vi "Camera Get Image.vi"(5 "Xmit":bool, 7 "Network Data":T2, 8 "error in (no error)":errorcluster, 9 "Camera Cluster":cluster{"Session Out":T4, "Camera Number":i32}, 10 "Camera Controls":T5 {"VideoMode" items=["640 x 480 YUY 2 30.00 fps", "640 x 480 YUY 2 20.00 fps", "640 x 480 YUY 2 15.00 fps", "640 x 480 YUY 2 10.00 fps", "640 x 480 YUY 2 7.50 fps", "1280 x 720 YUY 2 10.00 fps", "1280 x 720 YUY 2 7.50 fps", "960 x 544 YUY 2 15.00 fps", "960 x 544 YUY 2 10.00 fps", "960 x 544 YUY 2 7.50 fps", "800 x 448 YUY 2 20.00 fps", "800 x 448 YUY 2 15.00 fps", "800 x 448 YUY 2 10.00 fps", "800 x 448 YUY 2 7.50 fps", "640 x 360 YUY 2 30.00 fps", "640 x 360 YUY 2 20.00 fps", "640 x 360 YUY 2 15.00 fps", "640 x 360 YUY 2 10.00 fps", "640 x 360 YUY 2 7.50 fps", "424 x 240 YUY 2 30.00 fps", "424 x 240 YUY 2 20.00 fps", "424 x 240 YUY 2 15.00 fps", "424 x 240 YUY 2 10.00 fps", "424 x 240 YUY 2 7.50 fps", "352 x 288 YUY 2 30.00 fps", "352 x 288 YUY 2 20.00 fps", "352 x 288 YUY 2 15.00 fps", "352 x 288 YUY 2 10.00 fps", "352 x 288 YUY 2 7.50 fps", "320 x 240 YUY 2 30.00 fps", "320 x 240 YUY 2 20.00 fps", "320 x 240 YUY 2 15.00 fps", "320 x 240 YUY 2 10.00 fps", "320 x 240 YUY 2 7.50 fps", "800 x 600 YUY 2 15.00 fps", "800 x 600 YUY 2 10.00 fps", "800 x 600 YUY 2 7.50 fps", "176 x 144 YUY 2 30.00 fps", "176 x 144 YUY 2 20.00 fps", "176 x 144 YUY 2 15.00 fps", "176 x 144 YUY 2 10.00 fps", "176 x 144 YUY 2 7.50 fps", "160 x 120 YUY 2 30.00 fps", "160 x 120 YUY 2 20.00 fps", "160 x 120 YUY 2 15.00 fps", "160 x 120 YUY 2 10.00 fps", "160 x 120 YUY 2 7.50 fps", "1280 x 800 YUY 2 10.00 fps", "640 x 480 JPEG 30.00 fps", "640 x 480 JPEG 20.00 fps", "640 x 480 JPEG 15.00 fps", "640 x 480 JPEG 10.00 fps", "640 x 480 JPEG 7.50 fps", "1280 x 720 JPEG 30.00 fps", "1280 x 720 JPEG 20.00 fps", "1280 x 720 JPEG 15.00 fps", "1280 x 720 JPEG 10.00 fps", "1280 x 720 JPEG 7.50 fps", "960 x 544 JPEG 30.00 fps", "960 x 544 JPEG 20.00 fps", "960 x 544 JPEG 15.00 fps", "960 x 544 JPEG 10.00 fps", "960 x 544 JPEG 7.50 fps", "800 x 448 JPEG 30.00 fps", "800 x 448 JPEG 20.00 fps", "800 x 448 JPEG 15.00 fps", "800 x 448 JPEG 10.00 fps", "800 x 448 JPEG 7.50 fps", "640 x 360 JPEG 30.00 fps", "640 x 360 JPEG 20.00 fps", "640 x 360 JPEG 15.00 fps", "640 x 360 JPEG 10.00 fps", "640 x 360 JPEG 7.50 fps", "800 x 600 JPEG 30.00 fps", "800 x 600 JPEG 20.00 fps", "800 x 600 JPEG 15.00 fps", "800 x 600 JPEG 10.00 fps", "800 x 600 JPEG 7.50 fps", "416 x 240 JPEG 30.00 fps", "416 x 240 JPEG 20.00 fps", "416 x 240 JPEG 15.00 fps", "416 x 240 JPEG 10.00 fps", "416 x 240 JPEG 7.50 fps", "352 x 288 JPEG 30.00 fps", "352 x 288 JPEG 20.00 fps", "352 x 288 JPEG 15.00 fps", "352 x 288 JPEG 10.00 fps", "352 x 288 JPEG 7.50 fps", "176 x 144 JPEG 30.00 fps", "176 x 144 JPEG 20.00 fps", "176 x 144 JPEG 15.00 fps", "176 x 144 JPEG 10.00 fps", "176 x 144 JPEG 7.50 fps", "320 x 240 JPEG 30.00 fps", "320 x 240 JPEG 20.00 fps", "320 x 240 JPEG 15.00 fps", "320 x 240 JPEG 10.00 fps", "320 x 240 JPEG 7.50 fps", "160 x 120 JPEG 30.00 fps", "160 x 120 JPEG 20.00 fps", "160 x 120 JPEG 15.00 fps", "160 x 120 JPEG 10.00 fps", "160 x 120 JPEG 7.50 fps"]}, 11 "Refnum in":T1) -> (3 "Refnum out":T1(plugin-control))   [LabVIEW 2016]
uses:
  Camera Settings.ctl
  38 Video Mode.ctl
  <vilib>/userdefined/High Color/IMAQdx.ctl
  TCP Port Control.ctl
  <vilib>/vision/Image Controls.llb/IMAQ Image.ctl
  <vilib>/vision/driver/IMAQdx.llb/IMAQdx Buffer Number Mode.ctl
  <vilib>/vision/driver/NI_Vision_Acquisition_Software.lvlib
  <resource>/objmgr/imaqdx.rc
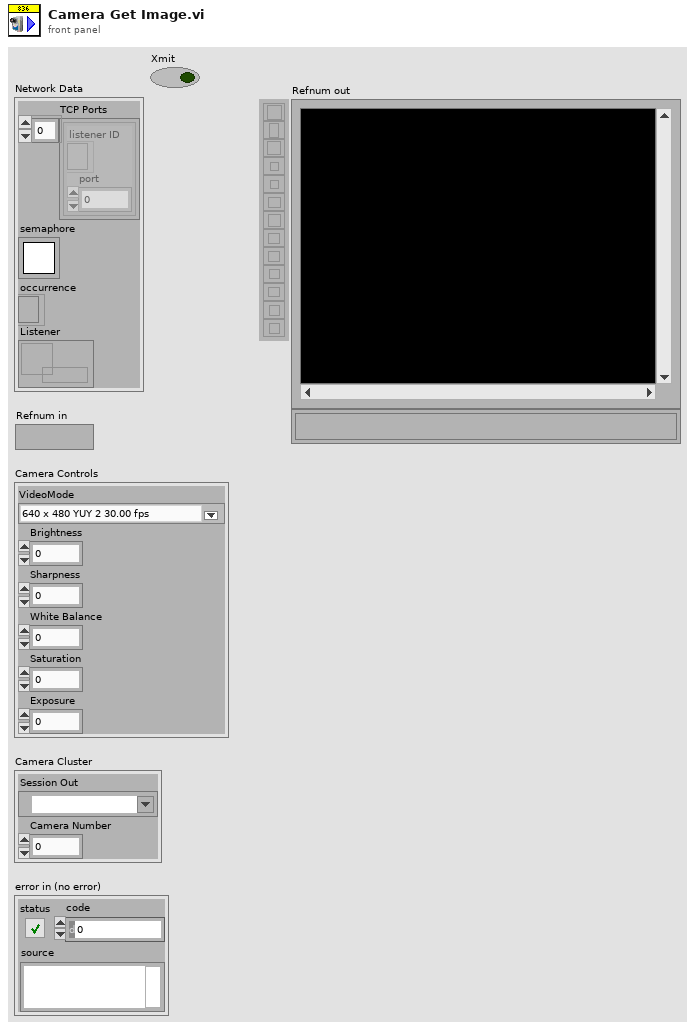
[diagram p1: front panel]
types:
  T1 = typedef "IMAQ Image.ctl" = refnum<image>
  T2 = typedef "TCP Port Control.ctl" = cluster{"TCP Ports":cluster{"listener ID":refnum<k5>, "port":u16}[], "semaphore":T3, "occurrence":refnum<k4>, "Listener":refnum<data-value>}
  T3 = typedef "Semaphore RefNum" = refnum<k1>
  T4 = typedef "IMAQdx.ctl" = refnum<k21>
  T5 = typedef "Camera Settings.ctl" = cluster{"VideoMode":T6, "Brightness":i64, "Sharpness":i64, "White Balance":i64, "Saturation":i64, "Exposure":i64}
  T6 = typedef "38 Video Mode.ctl" = u32
  T7 = typedef "NI_Vision_Acquisition_Software.lvlib/IMAQdx Buffer Number Mode.ctl" = enum32{"Next", "Last", "Buffer Number", "Every", "Last New"}
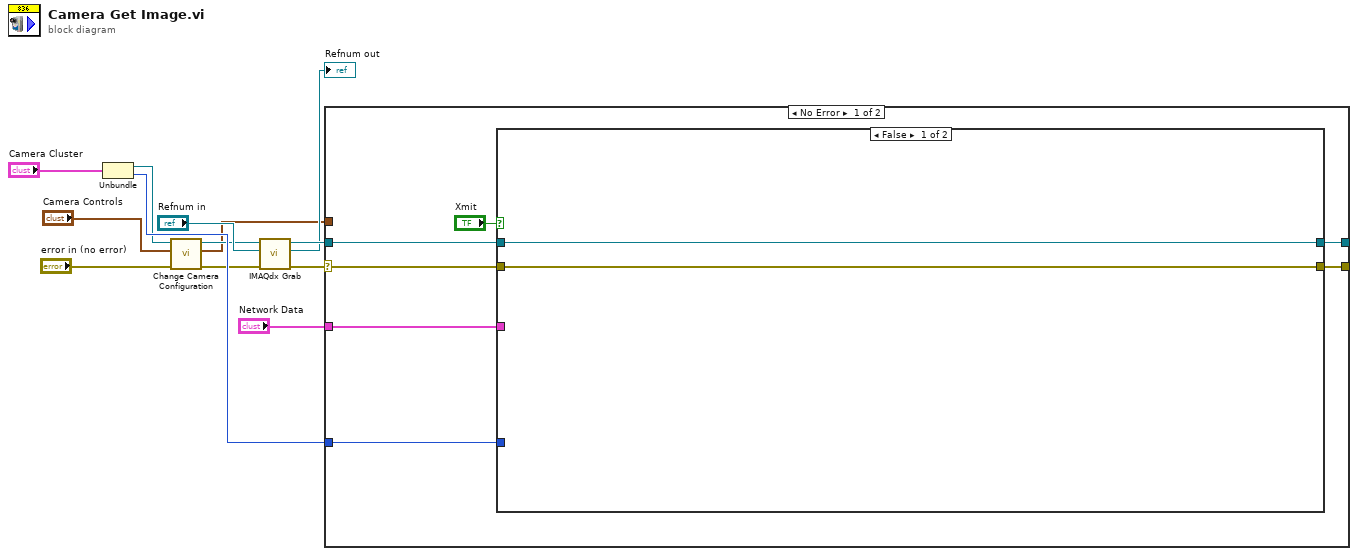
[diagram p0: block diagram]
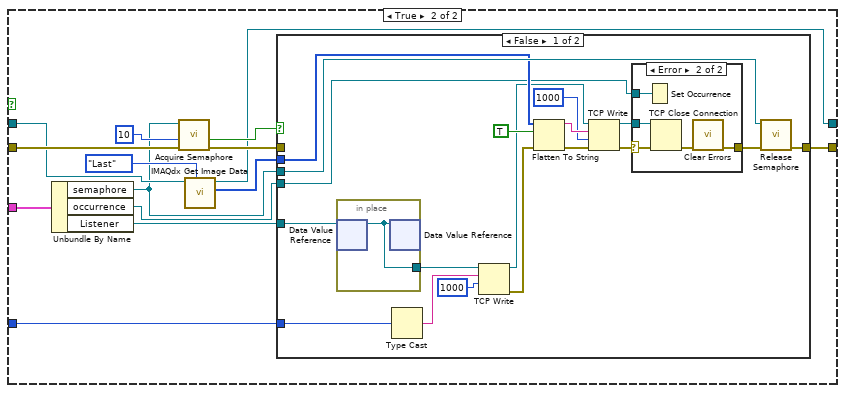
[diagram p2: hidden frame]
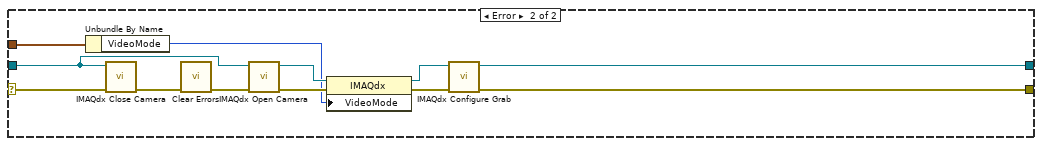
[diagram p5: hidden frame]
diagram:
  n1 = Unbundle("Camera Cluster") -> ("Session Out"=w10:T4, "Camera Number"=w11:i32)
  n2 = call "Change Camera Configuration.vi"("error in (no error)"="error in (no error)", "Camera Controls"="Camera Controls", "Camera Session"=w10) -> ("error out"=w5:errorcluster, "Camera Controls Out"=w1:T5, "Session out"=w2:T4)  [unwired: 6 in]
  n3 = call <vilib>:"IMAQdx Grab.vi"("error in"=w5, "Image In"="Refnum in", "Session In"=w2) -> ("error out"=w6:errorcluster, "Image Out"=→"Refnum out":T1, "Session Out"=w7:T4)  [unwired: 5 in, 1 out]
  n4 = case shown="No Error" w6 {
    selector: w6 -> [w19 w69]
    tunnel: w11 -> [w20 _]
    tunnel: w7 -> [w17 w68]
    tunnel: [w18 w67] -> _
    tunnel: [w16 w66] -> _
    tunnel: w1 -> [_ w63]
    tunnel: "Network Data" -> [w15 _]
    frame No Error {
      n5 = case shown="False" "Xmit" {
        tunnel: w20 -> [_ w34]
        tunnel: w19 -> [w21 w33]
        tunnel: [w21 w32] -> w18
        tunnel: w17 -> [w22 w30]
        tunnel: [w22 w29] -> w16
        tunnel: w15 -> [_ w23]
        frame False {
        }
        frame True {
          n6 = Unbundle By Name(w23) -> ("semaphore"=w24:T3, "occurrence"=w26:refnum<k4>, "Listener"=w25:refnum<data-value>)
          n7 = call <vilib>:"Acquire Semaphore.vi"("error in (no error)"=w33, "ms timeout (-1)"=10, "semaphore"=w24) -> ("error out"=w31:errorcluster, "timed out"=w36:bool)  [unwired: 2 in, 1 out]
          n8 = call <vilib>:"IMAQdx Get Image Data.vi"("Buffer Number Mode (Next)"=IMAQdx_Buffer_Number_Mode."Last", "Session In"=w30) -> ("Image Data Array"=w28:u8[], "Session Out"=w29:T4)  [unwired: 6 in, 2 out]
          n9 = case shown="False" w36 {
            tunnel: w24 -> [w50 _]
            tunnel: w25 -> [w49 _]
            tunnel: w28 -> [w47 _]
            tunnel: w34 -> [w46 _]
            tunnel: w26 -> [w41 _]
            tunnel: [w39 _] -> w32
            tunnel: w31 -> [_ _]
            frame False {
              n10 = in-place {
                in-place-border: [w61] -> w48
                n11 = in-place-dvr #1(w49) -> (w61:refnum<k5>)  [unwired: 1 out]
                n12 = in-place-dvr #1(w61) -> ()  [unwired: 2 out]
              }
              n13 = Type Cast(x=w46) -> (*(type *) &x=w45:string)  [unwired: 1 in]
              n14 = TCP Write(connection ID=w48, data in=w45, 9:1000 ("timeout ms (25000)")) -> (connection ID out=w38:refnum<k5>, error out=w51:errorcluster)  [unwired: 1 in, 1 out]
              n15 = Flatten To String(anything=w47, prepend array or string size? (T)=TRUE, error in (no error)=w51) -> (data string=w53:string, error out=w54:errorcluster)  [unwired: 1 in, 1 out]
              n16 = TCP Write(connection ID=w38, data in=w53, error in (no error)=w54, 9:1000 ("timeout ms (25000)")) -> (connection ID out=w37:refnum<k5>, error out=w42:errorcluster)  [unwired: 1 out]
              n17 = case shown="Error" w42 {
                selector: w42 -> [w55 w58]
                tunnel: w41 -> [_ w60]
                tunnel: [w55 w56] -> w40
                tunnel: w37 -> [_ w59]
                frame No Error {
                }
                frame Error {
                  n18 = Set Occurrence(w60) -> ()
                  n19 = TCP Close Connection(connection ID=w59, error in (no error)=w58) -> (error out=w57:errorcluster)  [unwired: 1 in, 1 out]
                  n20 = call <vilib>:"Clear Errors.vi"("error in (no error)"=w57) -> ("error out"=w56:errorcluster)  [unwired: 5 in, 1 out]
                }
              }
              n21 = call <vilib>:"Release Semaphore.vi"("error in (no error)"=w40, "semaphore"=w50) -> ("error out"=w39:errorcluster)  [unwired: 4 in, 1 out]
            }
            frame True {
            }
          }
        }
      }
    }
    frame Error {
      n22 = Unbundle By Name(w63) -> ("VideoMode"=w62:T6)
      n23 = call <vilib>:"IMAQdx Close Camera.vi"("error in"=w69, "Session In"=w68) -> ("error out"=w73:errorcluster)  [unwired: 9 in]
      n24 = call <vilib>:"Clear Errors.vi"("error in (no error)"=w73) -> ("error out"=w72:errorcluster)  [unwired: 5 in, 1 out]
      n25 = call <vilib>:"IMAQdx Open Camera.vi"("error in"=w72, "Session In"=w68) -> ("error out"=w71:errorcluster, "Session Out"=w65:T4)  [unwired: 8 in]
      n26 = property class="IMAQdx"(reference=w65, error in=w71, "VideoMode"=w62) -> (reference out=w64:T4, error out=w70:errorcluster)
      n27 = call <vilib>:"IMAQdx Configure Grab.vi"("error in"=w70, "Session In"=w64) -> ("error out"=w67:errorcluster, "Session Out"=w66:T4)  [unwired: 8 in]
    }
  }
